vi "DecodificaDO.vi"(0 "Array":T7[](array[typedef]), 7 "DO PLCs in":T5, 9 "statoDO Cdaq in":T9, 11 "DO interfaccia in":T6) -> (6 "Exit?":bool, 8 "DO PLCs out":T4, 10 "statoDO Cdaq out":T9, 15 "DO interfaccia out":T6)   [LabVIEW 2019]
uses:
  controls/statoDO_Cdaq.ctl
  SET SINGLE DO.ctl
  DO List.ctl
  TypeDef/DOinterfaccia.ctl
  ST1200_LIST_IO/StatoDO_PLC_1.ctl
  ST1200_LIST_IO/StatoDO_PLC_2.ctl
  ST1200_LIST_IO/StatoDO_PLC_3.ctl
  GlobalForzaUscite.vi
  Global_DO_Interfaccia.vi
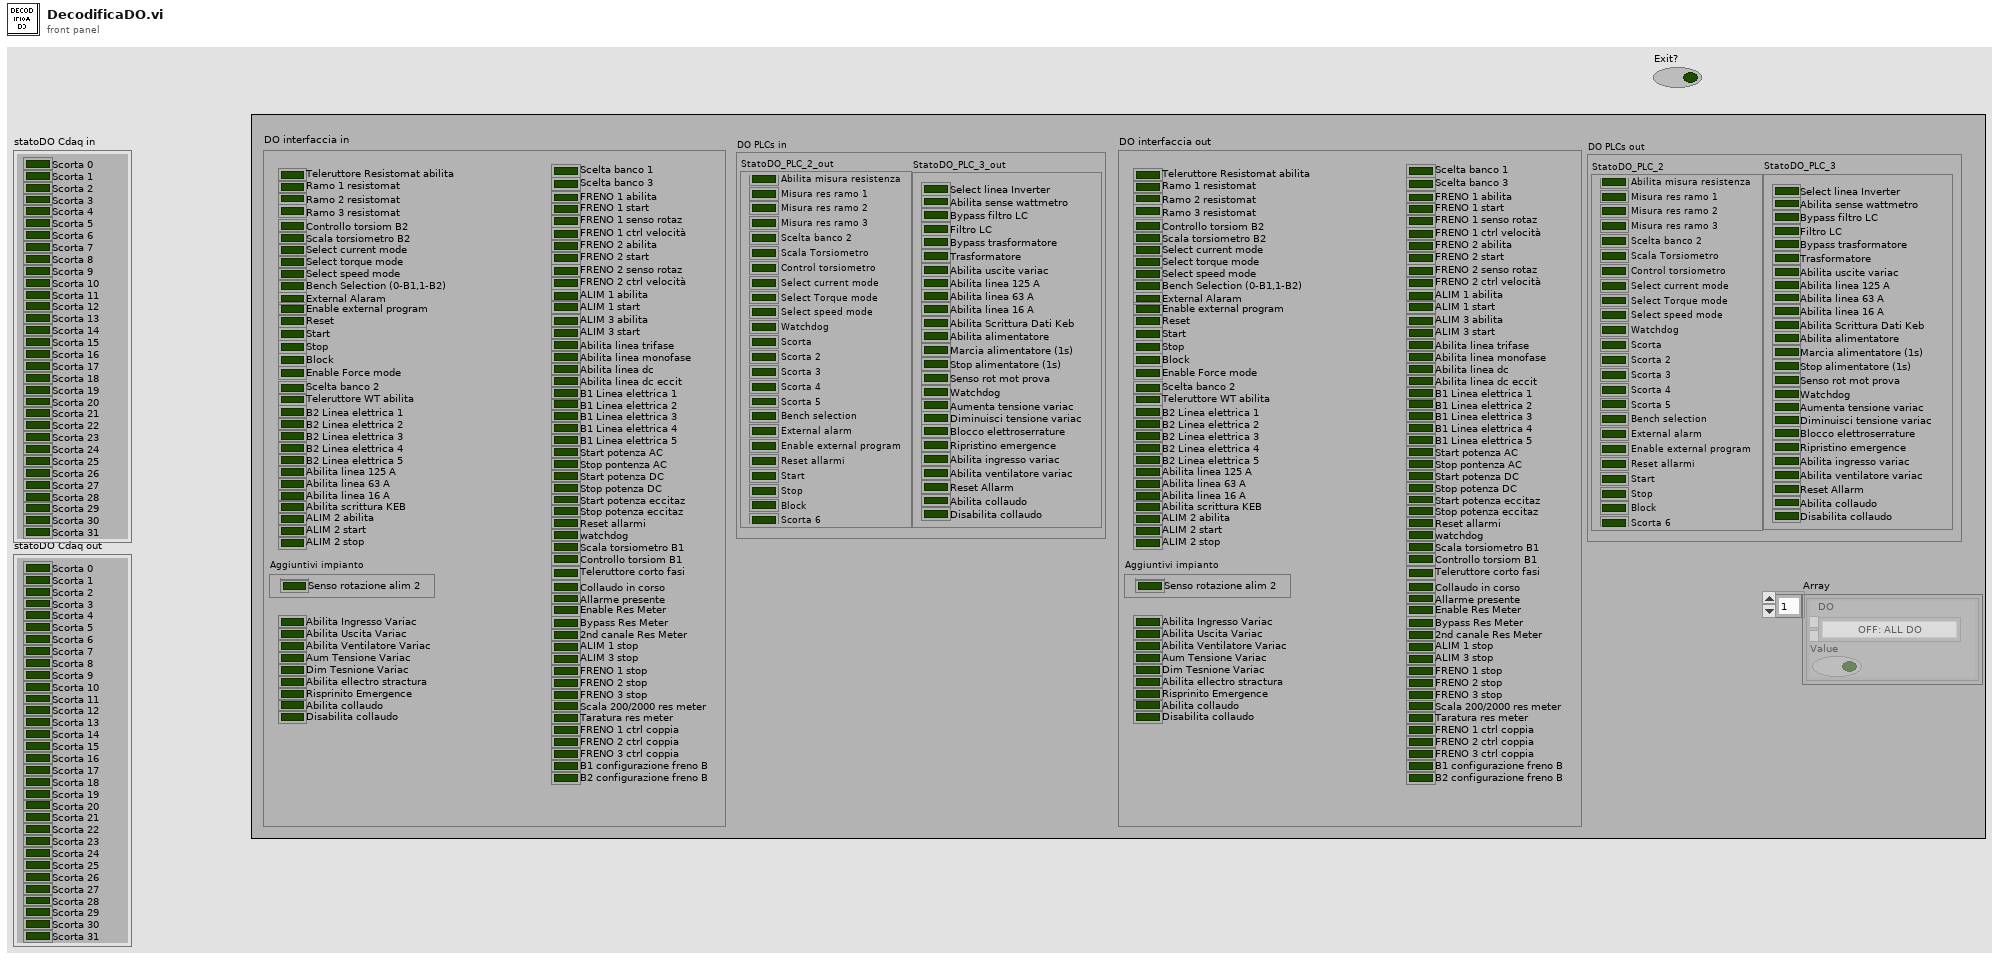
[diagram p1: front panel]
types:
  T1 = typedef "StatoDO_PLC_1.ctl" = cluster{"Scelta banco 1":bool, "Set dati motore freno 2":bool, "Diretto inverter":bool, "Filtro LC":bool, "Marcia ALIM (1s)":bool, "Marcia FRENO (1s)":bool, "Stop AFE (1s)":bool, "Stop freno (1s)":bool, "Reset allarmi":bool, "Watchdog":bool, "Senso rotazione":bool, "Abilita collaudo (1s)":bool, "Disabilita collaudo (1s)":bool, "Abilitazione ALIM":bool, "Abilitazione FRENO":bool, "Teleruttore WT":bool, "Senso rot motore prova":bool, "Scorta 7":bool, "Scorta 8":bool, "Scorta 9":bool, "Scorta 10":bool, "Scorta 11":bool, "Scorta 12":bool, "Scorta 13":bool}
  T2 = typedef "StatoDO_PLC_2.ctl" = cluster{"Relè misura resistomat":bool, "Misura res ramo 1":bool, "Misura res ramo 2":bool, "Misura res ramo 3":bool, "Scelta banco 2":bool, "Scala Torsiometro":bool, "Ctrl torsiometro":bool, "Select current mode":bool, "Select Torque mode":bool, "Select speed mode":bool, "Watchdog":bool, "Scorta":bool, "Scorta 2":bool, "Scorta 3":bool, "Scorta 4":bool, "Scorta 5":bool, "Bench selection":bool, "External alarm":bool, "Enable external program":bool, "Reset allarmi":bool, "Start":bool, "Stop":bool, "Block":bool, "Scorta 6":bool}
  T3 = typedef "StatoDO_PLC_3.ctl" = cluster{"Select linea Inverter":bool, "Abilita sense wattmetro":bool, "Bypass filtro LC":bool, "Filtro LC":bool, "Bypass trasformatore":bool, "Trasformatore":bool, "Abilita uscite variac":bool, "Abilita linea 125 A":bool, "Abilita linea 63 A":bool, "Abilita linea 16 A":bool, "Abilita Scrittura Dati Keb":bool, "Abilita alimentatore":bool, "Marcia alimentatore (1s)":bool, "Stop alimentatore (1s)":bool, "Senso rot mot prova":bool, "Watchdog":bool, "Aumenta tensione variac":bool, "Diminuisci tensione variac ":bool, "Blocco elettroserrature":bool, "Ripristino emergence":bool, "Abilita ingresso variac":bool, "Abilita ventilatore variac":bool, "Reset Allarm":bool, "Scorta 1":bool, "Scorta 2":bool, "Scorta 3":bool, "Scorta 4":bool, "Scorta 5":bool, "Scorta 6":bool, "Scorta 7":bool, "Scorta 8":bool, "Scorta 9":bool, "Abilita collaudo":bool, "Disabilita collaudo ":bool, "Scorta 10":bool, "Scorta 11":bool, "Scorta 12":bool, "Scorta 13":bool, "Scorta 14":bool, "Scorta 15":bool}
  T4 = cluster{"StatoDO_PLC 1":T1, "StatoDO_PLC_2":T2, "StatoDO_PLC_3":T3}
  T5 = cluster{"StatoDO_PLC 1 in":T1, "StatoDO_PLC_2_out":T2, "StatoDO_PLC_3_out":T3}
  T6 = typedef "DOinterfaccia.ctl" = cluster{"Scelta banco 1":bool, "Scelta banco 2":bool, "Scelta banco 3":bool, "FRENO 1 abilita":bool, "FRENO 1 start":bool, "FRENO 1 senso rotaz":bool, "FRENO 1 ctrl velocità":bool, "FRENO 2 abilita":bool, "FRENO 2 start":bool, "FRENO 2 senso rotaz":bool, "FRENO 2 ctrl velocità":bool, "ALIM 1 abilita":bool, "ALIM 1 start":bool, "ALIM 2 abilita":bool, "ALIM 2 start":bool, "ALIM 3 abilita":bool, "ALIM 3 start":bool, "Abilita linea trifase":bool, "Abilita linea monofase":bool, "Abilita linea dc":bool, "Abilita linea dc eccit":bool, "B1 Linea elettrica 1":bool, "B1 Linea elettrica 2":bool, "B1 Linea elettrica 3":bool, "B1 Linea elettrica 4":bool, "B1 Linea elettrica 5":bool, "B2 Linea elettrica 1":bool, "B2 Linea elettrica 2":bool, "B2 Linea elettrica 3":bool, "B2 Linea elettrica 4":bool, "B2 Linea elettrica 5":bool, "Start potenza AC":bool, "Stop pontenza AC":bool, "Start potenza DC":bool, "Stop potenza DC":bool, "Start potenza eccitaz":bool, "Stop potenza eccitaz":bool, "Reset allarmi":bool, "watchdog":bool, "Scala torsiometro B1":bool, "Controllo torsiom B1":bool, "Scala torsiometro B2":bool, "Controllo torsiom B2":bool, "Teleruttore WT abilita":bool, "Teleruttore Resistomat abilita":bool, "Teleruttore corto fasi":bool, "Ramo 1 resistomat":bool, "Ramo 2 resistomat":bool, "Ramo 3 resistomat":bool, "Collaudo in corso":bool, "Allarme presente":bool, "Enable Res Meter":bool, "Bypass Res Meter":bool, "2nd canale Res Meter":bool, "Scala 200/2000 res meter":bool, "Taratura res meter":bool, "FRENO 1 ctrl coppia":bool, "FRENO 2 ctrl coppia":bool, "FRENO 3 ctrl coppia":bool, "Aggiuntivi impianto":cluster{"Senso rotazione alim 1":bool, "Senso rotazione alim 2":bool}, "ALIM 1 stop":bool, "ALIM 2 stop":bool, "ALIM 3 stop":bool, "FRENO 1 stop":bool, "FRENO 2 stop":bool, "FRENO 3 stop":bool, "B1 configurazione freno B":bool, "B2 configurazione freno B":bool, "Abilita scrittura KEB":bool, "Bench Selection (0-B1,1-B2)":bool, "Select current mode":bool, "Select torque mode":bool, "Select speed mode":bool, "Start":bool, "Stop":bool, "Block":bool, "Enable Force mode":bool, "Abilita linea 125 A":bool, "Abilita linea 63 A":bool, "Abilita linea 16 A":bool, "Aum Tensione Variac":bool, "Dim Tesnione Variac":bool, "Abilita ellectro stractura":bool, "Risprinito Emergence":bool, "Abilita collaudo":bool, "Disabilita collaudo":bool, "External Alaram":bool, "Enable external program":bool, "Reset":bool, "Abilita Ingresso Variac":bool, "Abilita Ventilatore Variac":bool, "Abilita Uscita Variac ":bool}
  T7 = typedef "SET SINGLE DO.ctl" = cluster{"DO":T8, "Value":bool}
  T8 = typedef "DO List.ctl" = enum16{"OFF: ALL DO", "*ABILITA freno 1", "*ABILITA freno 2", "*ABILITA freno 3", "*START freno 1", "*START freno 2", "*START freno 3", "*STOP freno 1", "*STOP freno 3", "*STOP freno 2", "*Senso rot freno 1", "*Senso rot freno 2", "*Senso rot freno 3", "*Ctrl velocità freno 1", "*Ctrl velocità freno 2", "*Ctrl velocità freno 3", "*Ctrl coppia freno 1", "*Ctrl coppia freno 2", "*Ctrl coppia freno 3", "*ABILITA alimentatore 1", "*ABILITA alimentatore 2", "*ABILITA alimentatore 3", "*ABILITA alimentatore 4", "*START alimentatore 1", "*START alimentatore 2", "*START alimentatore 3", "*START alimentatore 4", "*STOP alimentatore 1", "*STOP alimentatore 2", "*STOP alimentatore 3", "*STOP alimentatore 4", "SENSO ROT alimentatore 1", "SENSO ROT alimentatore 2", "Abilita LEM 1000A", "Abilita LEM 300A", "Abilita sensori EXT WT", "B1 Seleziona linea 1", "B1 Seleziona linea 2", "B1 Seleziona linea 3", "B1 Seleziona linea 4", "B1 Seleziona linea 5", "B2 Seleziona linea 1", "B2 Seleziona linea 2", "B2 Seleziona linea 3", "B2 Seleziona linea 4", "B2 Seleziona linea 5", "*Reset allarmi", "*Start potenza AC", "*Stop potenza AC", "*Start potenza DC", "*Stop potenza DC", "*Start potenza DC eccit", "*Stop pontenza DC eccit", "Bypass res meter", "2nd canale res meter", "Enable res meter", "*Abilit teler ramo WT", "*Abil teler ramo princ Resit", "*Abil teler ramo 1 Resist", "*Abil teler ramo 2 Resist", "*Abil teler ramo 3 Resist", "*Abil cortocirc avvolgim", "*Controllo torsiometro B1", "*Controllo Torsiom B2", "*Scala torsiometro B1", "*Scala torsiometro B2", "*Collaudo in corso", "*Allarme presente", "Abilitazione elettroserratura", "Exit", "*Abilita collaudo", "*Abilita potenza trifase", "*Abilita potenza monofase", "*Abilita potenza DC", "*Abilita potenza DC eccit", "*Disabilita teleruttori potenza", "Set teleruttori prova a freddo", "Prova a freddo monofase", "Watchdog", "Forza DO PLC 3", "Forza DO PLC 2", "Forza DO PLC 1", "Forza DO cDAQ", "Scala 2000(T) 200(F) res meter", "Seleziona banco 1", "Seleziona banco 2", "Comando azionam in blocco", "Comando azionam reset", "Sensibilità freno 16 32 nm", "Reset Allarmi", "Carico res - Ramo 1", "Carico res - Ramo 2", "Carico res - Ramo 3", "Carico res - Ramo 4", "Carico res - Ramo 5", "Carico res - Ramo 6", "Carico res - Ramo 7", "Carico res - Ramo 8", "Carico res - Ramo 9", "Carico res - Ramo 10", "Carico res - Ramo 11", "Carico res - Start ventilatore", "Carico res - Stop ventilatore", "Abilita potenza solo freno", "Abilita AFE + freno trasc", "Abilita potenza carico resistivo", "Chiudi potenza AFE", "Apri potenza AFE", "Start AFE", "Config Banco2 TDE", "Misura diretto WT", "Ripristina centralina protezioni", "Abilita Scrittura Dati Keb", "Bench Selection(0-B1,1-B2)", "Select current mode", "Select torque mode", "Select speed mode", "Extenal alarm", "Enable Extenal program ", "Start ", "Stop", "Enable force mode", "Abilita linea 125 A", "Abilita linea 63 A", "Abilita linea 16 A", "Aum Tensione Variac", "Dim Tesnione Variac", "Abilita Ellecto Stractura", "Riprinto Emergenxe ", "Abilita Collaudo", "Disabilita Collaudo", "Abilita Ingresso Variac", "Abilita Uscita Variac", "Abilita ventilatore Variac"}
  T9 = typedef "statoDO_Cdaq.ctl" = cluster{"Scorta 0":bool, "Scorta 1":bool, "Scorta 2":bool, "Scorta 3":bool, "Scorta 4":bool, "Scorta 5":bool, "Scorta 6":bool, "Scorta 7":bool, "Scorta 8":bool, "Scorta 9":bool, "Scorta 10":bool, "Scorta 11":bool, "Scorta 12":bool, "Scorta 13":bool, "Scorta 14":bool, "Scorta 15":bool, "Scorta 16":bool, "Scorta 17":bool, "Scorta 18":bool, "Scorta 19":bool, "Scorta 20":bool, "Scorta 21":bool, "Scorta 22":bool, "Scorta 23":bool, "Scorta 24":bool, "Scorta 25":bool, "Scorta 26":bool, "Scorta 27":bool, "Scorta 28":bool, "Scorta 29":bool, "Scorta 30":bool, "Scorta 31":bool}
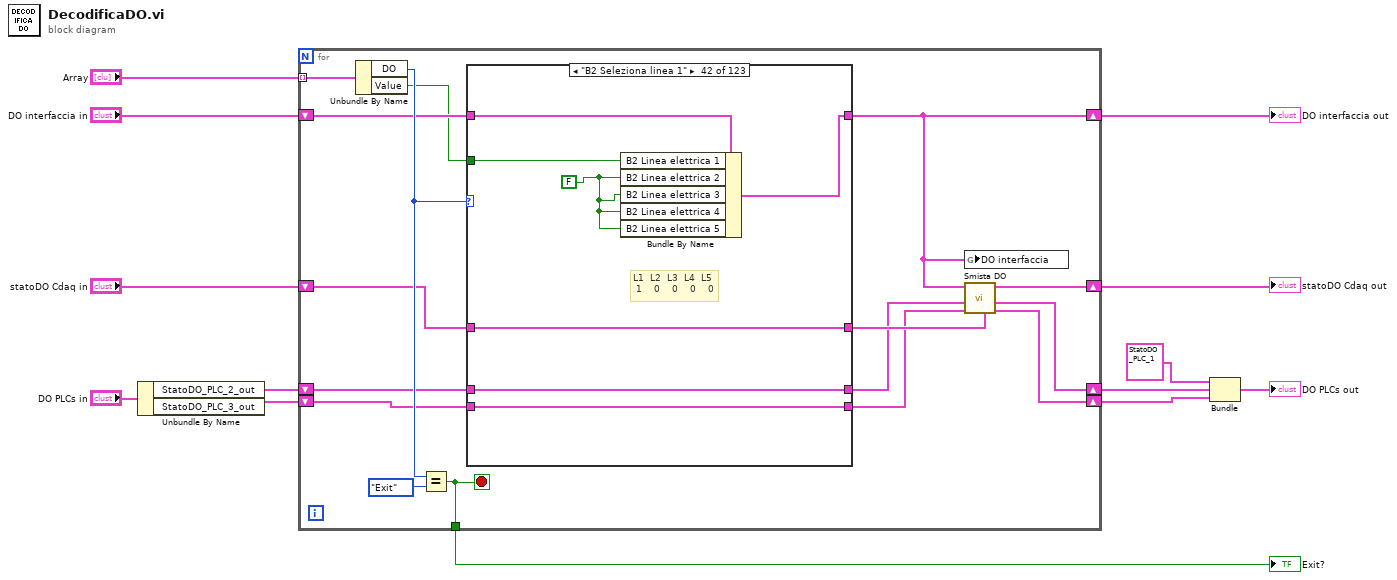
[diagram p0: block diagram]
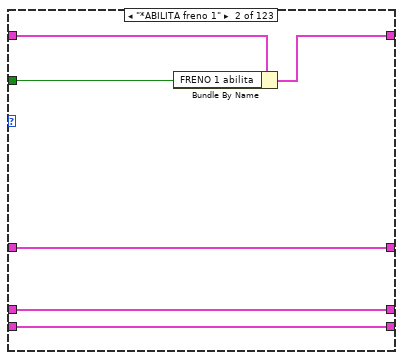
[diagram p3: hidden frame]
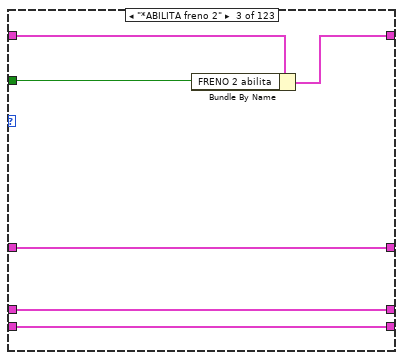
[diagram p4: hidden frame]
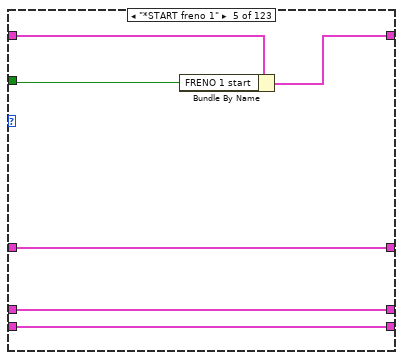
[diagram p6: hidden frame]
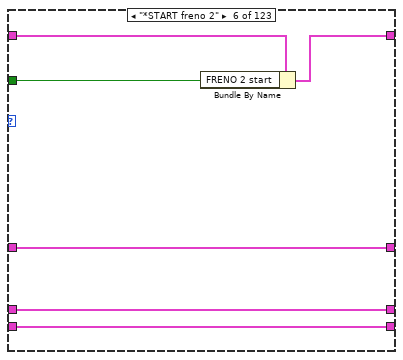
[diagram p7: hidden frame]
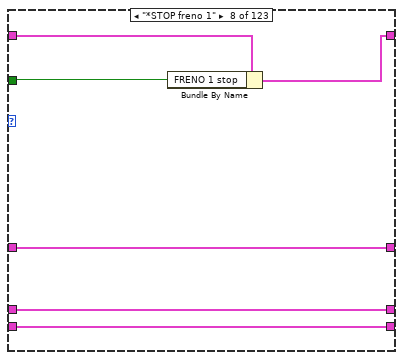
[diagram p9: hidden frame]
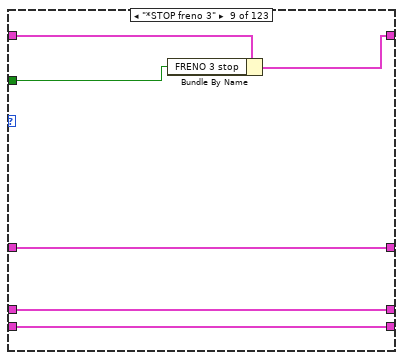
[diagram p10: hidden frame]
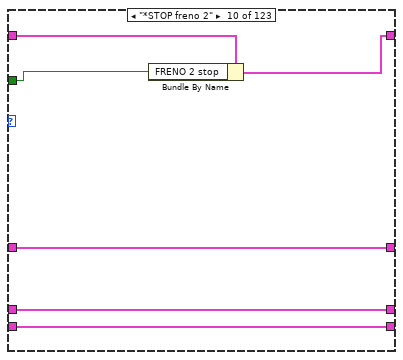
[diagram p11: hidden frame]
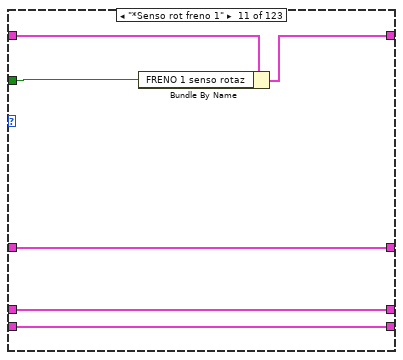
[diagram p12: hidden frame]
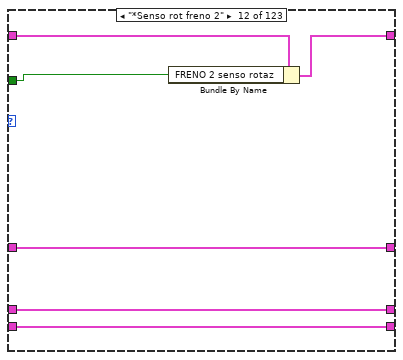
[diagram p13: hidden frame]
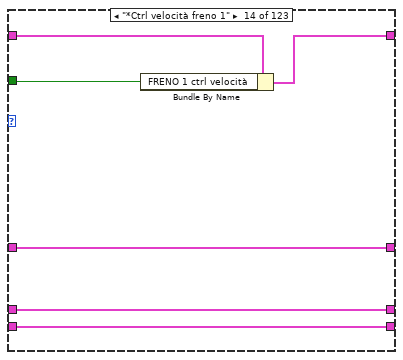
[diagram p15: hidden frame]
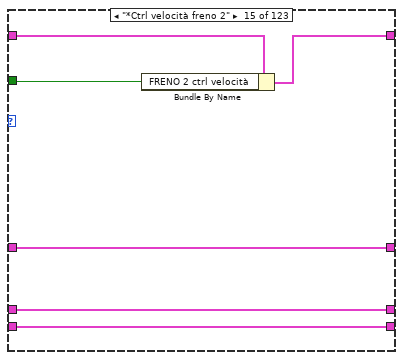
[diagram p16: hidden frame]
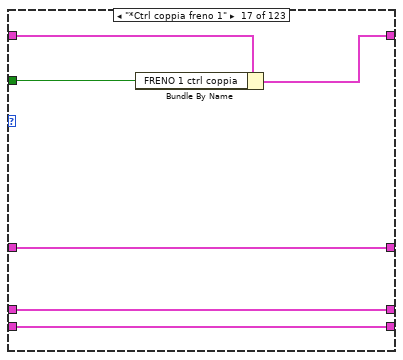
[diagram p18: hidden frame]
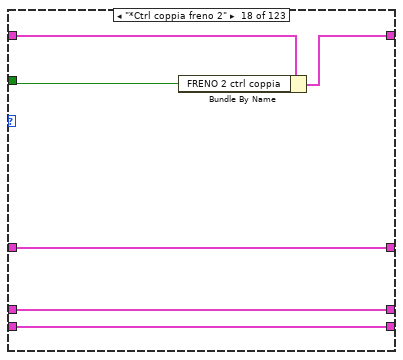
[diagram p19: hidden frame]
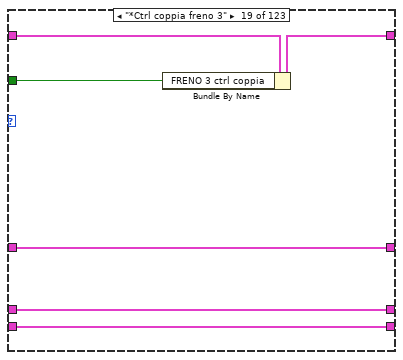
[diagram p20: hidden frame]
diagram:
  n1 = Unbundle By Name("DO PLCs in") -> ("StatoDO_PLC_2_out"=w6:T2, "StatoDO_PLC_3_out"=w5:T3)
  n2 = for {
    tunnel: "Array" -> [w29] mode=indexing
    shift-right: [w26] -> w10
    shift-left: "statoDO Cdaq in" -> [w21]
    tunnel: [w28] -> w13
    shift-right: [w20] -> w8
    shift-left: "DO interfaccia in" -> [w23]
    shift-right: [w19] -> w4
    shift-left: w6 -> [w16]
    shift-right: [w18] -> w3
    shift-left: w5 -> [w17]
    stop <- w28 stop-if-true
    n3 = Unbundle By Name(w29) -> ("DO"=w25:T8, "Value"=w22:bool)
    n4 = Equal?(x=w25, y=DO_List."Exit" ("DO")) -> (x = y?=w28:bool)
    n5 = case shown="\"B2 Seleziona linea 1\"" w25 {
      tunnel: [w32 w38 w44 w48 w54 w60 w64 w70 w76 w82 w88 w94 w98 w104 w110 w114 w120 w126 w132 w138 w144 w150 w154 w160 w166 w172 w176 w182 w188 w194 w198 w204 w210 w216 w220 w224 w231 w238 w245 w252 w259 w266 w273 w280 w287 w294 w300 w306 w312 w318 w324 w328 w332 w338 w344 w350 w356 w362 w368 w374 w380 w386 w392 w398 w404 w410 w416 w422 w426 w430 w434 w441 w448 w455 w462 w468 w475 w479 w485 w487 w493 w497 w498 w507 w513 w519 w523 w527 w531 w537 w541 w545 w549 w553 w557 w561 w565 w569 w573 w577 w581 w585 w589 w595 w599 w603 w607 w611 w615 w621 w627 w631 w637 w643 w649 w655 w661 w667 w673 w679 w685 w691 w697] -> w24
      tunnel: [_ w35 w42 w47 w51 w58 w63 w65 w72 w78 w86 w92 w97 w102 w108 w113 w117 w124 w130 w136 w142 w148 w153 w158 w164 w170 w175 w177 w183 w189 w197 w200 w206 w211 w217 w221 w229 w235 w243 w250 w257 w262 w269 w276 w283 w290 w298 w304 w308 w316 w320 w325 w329 w336 w342 w348 w354 w360 w366 w372 w378 w384 w389 w396 w402 w407 w414 w420 w423 w429 w433 w439 w444 w451 w458 w466 w473 w478 w483 w489 w492 w496 w501 w505 w511 w515 w520 w524 w528 w535 w538 w542 w546 w550 w554 w558 w562 w566 w570 w574 w578 w582 w586 w591 w596 w600 w604 w608 w612 w617 w623 w628 w632 w638 w645 w651 w657 w663 w669 w675 w681 w687 w693] -> w20
      tunnel: w23 -> [_ w37 w43 w47 w52 w59 w63 w67 w73 w79 w87 w93 w97 w103 w109 w113 w118 w125 w131 w137 w143 w149 w153 w159 w165 w171 w175 w179 w184 w190 w197 w201 w207 w212 w217 w221 w230 w236 w244 w251 w258 w263 w270 w277 w284 w291 w299 w305 w309 w317 w321 w325 w329 w337 w343 w349 w355 w361 w367 w373 w379 w385 w390 w397 w403 w408 w415 w421 w423 w429 w433 w440 w445 w452 w459 w467 w474 w478 w484 w489 w492 w496 w501 w506 w512 w516 w520 w524 w528 w536 w538 w542 w546 w550 w554 w558 w562 w566 w570 w574 w578 w582 w586 w592 w596 w600 w604 w608 w612 w618 w624 w628 w634 w640 w646 w652 w658 w664 w670 w676 w682 w688 w694]
      tunnel: w22 -> [_ w36 w41 _ w53 w57 _ w66 w71 w77 w85 w91 _ w101 w107 _ w119 w123 w129 w135 w141 w147 _ w157 w163 w169 _ w178 w185 w191 _ w199 w205 w213 _ _ w228 w237 w242 w249 w256 w261 w268 w275 w282 w288 w295 w303 w307 w315 w319 _ _ w335 w341 w347 w353 w359 w365 w371 w377 w383 w391 w395 w401 w409 w413 w419 _ _ _ w438 w443 w450 w457 _ _ _ w482 _ _ _ _ w504 w510 w514 _ _ _ w532 _ _ _ _ _ _ _ _ _ _ _ _ _ _ _ _ _ _ _ w616 w622 _ w633 w639 w644 w650 w656 w662 w668 w674 w680 w686 w692]
      tunnel: w21 -> [w32 w38 w44 w48 w54 w60 w64 w70 w76 w82 w88 w94 w98 w104 w110 w114 w120 w126 w132 w138 w144 w150 w154 w160 w166 w172 w176 w182 w188 w194 w198 w204 w210 w216 w220 w224 w231 w238 w245 w252 w259 w266 w273 w280 w287 w294 w300 w306 w312 w318 w324 w328 w332 w338 w344 w350 w356 w362 w368 w374 w380 w386 w392 w398 w404 w410 w416 w422 w426 w430 w434 w441 w448 w455 w462 w468 w475 w479 w485 w487 w493 w497 _ w507 w513 w519 w523 w527 w531 w537 w541 w545 w549 w553 w557 w561 w565 w569 w573 w577 w581 w585 w589 w595 w599 w603 w607 w611 w615 w621 w627 w631 w637 w643 w649 w655 w661 w667 w673 w679 w685 w691 w697]
      tunnel: w17 -> [w30 w33 w39 w45 w49 w55 w61 w68 w74 w80 w83 w89 w95 w99 w105 w111 w115 w121 w127 w133 w139 w145 w151 w155 w161 w167 w173 w180 w186 w192 w195 w202 w208 w214 w218 w222 w225 w232 w239 w246 w253 w264 w271 w278 w285 w292 w296 w301 w310 w313 w322 w326 w330 w333 w339 w345 w351 w357 w363 w369 w375 w381 w387 w393 w399 w405 w411 w417 w424 w427 w431 w436 w446 w453 w460 w464 w469 w476 w480 _ w491 w494 w499 w502 w508 w517 w521 w525 w529 w533 w539 w543 w547 w551 w555 w559 w563 w567 w571 w575 w579 w583 w587 w593 w597 w601 w605 w609 w613 w619 w625 w629 w635 w641 w647 w653 w659 w665 w671 w677 w683 w689 w695]
      tunnel: w16 -> [w31 w34 w40 w46 w50 w56 w62 w69 w75 w81 w84 w90 w96 w100 w106 w112 w116 w122 w128 w134 w140 w146 w152 w156 w162 w168 w174 w181 w187 w193 w196 w203 w209 w215 w219 w223 w226 w233 w240 w247 w254 w265 w272 w279 w286 w293 w297 w302 w311 w314 w323 w327 w331 w334 w340 w346 w352 w358 w364 w370 w376 w382 w388 w394 w400 w406 w412 w418 w425 w428 w432 w437 w447 w454 w461 w465 w470 w477 w481 w488 _ w495 w500 w503 w509 w518 w522 w526 w530 w534 w540 w544 w548 w552 w556 w560 w564 w568 w572 w576 w580 w584 w588 w594 w598 w602 w606 w610 w614 w620 w626 w630 w636 w642 w648 w654 w660 w666 w672 w678 w684 w690 w696]
      tunnel: [w31 w34 w40 w46 w50 w56 w62 w69 w75 w81 w84 w90 w96 w100 w106 w112 w116 w122 w128 w134 w140 w146 w152 w156 w162 w168 w174 w181 w187 w193 w196 w203 w209 w215 w219 w223 w226 w233 w240 w247 w254 w265 w272 w279 w286 w293 w297 w302 w311 w314 w323 w327 w331 w334 w340 w346 w352 w358 w364 w370 w376 w382 w388 w394 w400 w406 w412 w418 w425 w428 w432 w437 w447 w454 w461 w465 w470 w477 w481 w488 w490 w495 w500 w503 w509 w518 w522 w526 w530 w534 w540 w544 w548 w552 w556 w560 w564 w568 w572 w576 w580 w584 w588 w594 w598 w602 w606 w610 w614 w620 w626 w630 w636 w642 w648 w654 w660 w666 w672 w678 w684 w690 w696] -> w15
      tunnel: [w30 w33 w39 w45 w49 w55 w61 w68 w74 w80 w83 w89 w95 w99 w105 w111 w115 w121 w127 w133 w139 w145 w151 w155 w161 w167 w173 w180 w186 w192 w195 w202 w208 w214 w218 w222 w225 w232 w239 w246 w253 w264 w271 w278 w285 w292 w296 w301 w310 w313 w322 w326 w330 w333 w339 w345 w351 w357 w363 w369 w375 w381 w387 w393 w399 w405 w411 w417 w424 w427 w431 w436 w446 w453 w460 w464 w469 w476 w480 w486 w491 w494 w499 w502 w508 w517 w521 w525 w529 w533 w539 w543 w547 w551 w555 w559 w563 w567 w571 w575 w579 w583 w587 w593 w597 w601 w605 w609 w613 w619 w625 w629 w635 w641 w647 w653 w659 w665 w671 w677 w683 w689 w695] -> w14
      frame "OFF: ALL DO", Default {
      }
      frame "*ABILITA freno 1" {
        n6 = Bundle By Name(cluster=w37, "FRENO 1 abilita"=w36) -> (w35:T6)
      }
      frame "*ABILITA freno 2" {
        n7 = Bundle By Name(cluster=w43, "FRENO 2 abilita"=w41) -> (w42:T6)
      }
      frame "*ABILITA freno 3" {
      }
      frame "*START freno 1" {
        n8 = Bundle By Name(cluster=w52, "FRENO 1 start"=w53) -> (w51:T6)
      }
      frame "*START freno 2" {
        n9 = Bundle By Name(cluster=w59, "FRENO 2 start"=w57) -> (w58:T6)
      }
      frame "*START freno 3" {
      }
      frame "*STOP freno 1" {
        n10 = Bundle By Name(cluster=w67, "FRENO 1 stop"=w66) -> (w65:T6)
      }
      frame "*STOP freno 3" {
        n11 = Bundle By Name(cluster=w73, "FRENO 3 stop"=w71) -> (w72:T6)
      }
      frame "*STOP freno 2" {
        n12 = Bundle By Name(cluster=w79, "FRENO 2 stop"=w77) -> (w78:T6)
      }
      frame "*Senso rot freno 1" {
        n13 = Bundle By Name(cluster=w87, "FRENO 1 senso rotaz"=w85) -> (w86:T6)
      }
      frame "*Senso rot freno 2" {
        n14 = Bundle By Name(cluster=w93, "FRENO 2 senso rotaz"=w91) -> (w92:T6)
      }
      frame "*Senso rot freno 3" {
      }
      frame "*Ctrl velocità freno 1" {
        n15 = Bundle By Name(cluster=w103, "FRENO 1 ctrl velocità"=w101) -> (w102:T6)
      }
      frame "*Ctrl velocità freno 2" {
        n16 = Bundle By Name(cluster=w109, "FRENO 2 ctrl velocità"=w107) -> (w108:T6)
      }
      frame "*Ctrl velocità freno 3" {
      }
      frame "*Ctrl coppia freno 1" {
        n17 = Bundle By Name(cluster=w118, "FRENO 1 ctrl coppia"=w119) -> (w117:T6)
      }
      frame "*Ctrl coppia freno 2" {
        n18 = Bundle By Name(cluster=w125, "FRENO 2 ctrl coppia"=w123) -> (w124:T6)
      }
      frame "*Ctrl coppia freno 3" {
        n19 = Bundle By Name(cluster=w131, "FRENO 3 ctrl coppia"=w129) -> (w130:T6)
      }
      frame "*ABILITA alimentatore 1" {
        n20 = Bundle By Name(cluster=w137, "ALIM 1 abilita"=w135) -> (w136:T6)
      }
      frame "*ABILITA alimentatore 2" {
        n21 = Bundle By Name(cluster=w143, "ALIM 2 abilita"=w141) -> (w142:T6)
      }
      frame "*ABILITA alimentatore 3" {
        n22 = Bundle By Name(cluster=w149, "ALIM 3 abilita"=w147) -> (w148:T6)
      }
      frame "*ABILITA alimentatore 4" {
      }
      frame "*START alimentatore 1" {
        n23 = Bundle By Name(cluster=w159, "ALIM 1 start"=w157) -> (w158:T6)
      }
      frame "*START alimentatore 2" {
        n24 = Bundle By Name(cluster=w165, "ALIM 2 start"=w163) -> (w164:T6)
      }
      frame "*START alimentatore 3" {
        n25 = Bundle By Name(cluster=w171, "ALIM 3 start"=w169) -> (w170:T6)
      }
      frame "*START alimentatore 4" {
      }
      frame "*STOP alimentatore 1" {
        n26 = Bundle By Name(cluster=w179, "ALIM 1 stop"=w178) -> (w177:T6)
      }
      frame "*STOP alimentatore 2" {
        n27 = Bundle By Name(cluster=w184, "ALIM 2 stop"=w185) -> (w183:T6)
      }
      frame "*STOP alimentatore 3" {
        n28 = Bundle By Name(cluster=w190, "ALIM 3 stop"=w191) -> (w189:T6)
      }
      frame "*STOP alimentatore 4" {
      }
      frame "SENSO ROT alimentatore 1" {
        n29 = Bundle By Name(cluster=w201, "Aggiuntivi impianto.Senso rotazione alim 1"=w199) -> (w200:T6)
      }
      frame "SENSO ROT alimentatore 2" {
        n30 = Bundle By Name(cluster=w207, "Aggiuntivi impianto.Senso rotazione alim 2"=w205) -> (w206:T6)
      }
      frame "Abilita LEM 1000A" {
        n31 = Bundle By Name(cluster=w212, "Aggiuntivi impianto.Senso rotazione alim 2"=w213) -> (w211:T6)
      }
      frame "Abilita LEM 300A" {
      }
      frame "Abilita sensori EXT WT" {
      }
      frame "B1 Seleziona linea 1" {
        w227 = FALSE ("Linea elettrica 5")
        n32 = Bundle By Name(cluster=w230, "B1 Linea elettrica 1"=w228, "B1 Linea elettrica 2"=w227, "B1 Linea elettrica 3"=w227, "B1 Linea elettrica 4"=w227, "B1 Linea elettrica 5"=w227) -> (w229:T6)
      }
      frame "B1 Seleziona linea 2" {
        w234 = FALSE ("Linea elettrica 1")
        n33 = Bundle By Name(cluster=w236, "B1 Linea elettrica 1"=w234, "B1 Linea elettrica 2"=w237, "B1 Linea elettrica 3"=w234, "B1 Linea elettrica 4"=w234, "B1 Linea elettrica 5"=w234) -> (w235:T6)
      }
      frame "B1 Seleziona linea 3" {
        w241 = FALSE ("Linea elettrica 1")
        n34 = Bundle By Name(cluster=w244, "B1 Linea elettrica 1"=w241, "B1 Linea elettrica 2"=w241, "B1 Linea elettrica 3"=w242, "B1 Linea elettrica 4"=w241, "B1 Linea elettrica 5"=w241) -> (w243:T6)
      }
      frame "B1 Seleziona linea 4" {
        w248 = FALSE ("Linea elettrica 5")
        n35 = Bundle By Name(cluster=w251, "B1 Linea elettrica 1"=w248, "B1 Linea elettrica 2"=w248, "B1 Linea elettrica 3"=w248, "B1 Linea elettrica 4"=w249, "B1 Linea elettrica 5"=w248) -> (w250:T6)
      }
      frame "B1 Seleziona linea 5" {
        w255 = FALSE ("Linea elettrica 1")
        n36 = Bundle By Name(cluster=w258, "B1 Linea elettrica 1"=w255, "B1 Linea elettrica 2"=w255, "B1 Linea elettrica 3"=w255, "B1 Linea elettrica 4"=w255, "B1 Linea elettrica 5"=w256) -> (w257:T6)
      }
      frame "B2 Seleziona linea 1" {
        w260 = FALSE
        # "L1  L2  L3  L4  L5\n 1    0    0    0    0"
        n37 = Bundle By Name(cluster=w263, "B2 Linea elettrica 1"=w261, "B2 Linea elettrica 2"=w260, "B2 Linea elettrica 3"=w260, "B2 Linea elettrica 4"=w260, "B2 Linea elettrica 5"=w260) -> (w262:T6)
      }
      frame "B2 Seleziona linea 2" {
        w267 = FALSE ("B1 Linea elettrica 2")
        # "L1  L2  L3  L4  L5\n 0    1    0    0    0"
        n38 = Bundle By Name(cluster=w270, "B2 Linea elettrica 1"=w267, "B2 Linea elettrica 2"=w268, "B2 Linea elettrica 3"=w267, "B2 Linea elettrica 4"=w267, "B2 Linea elettrica 5"=w267) -> (w269:T6)
      }
      frame "B2 Seleziona linea 3" {
        w274 = FALSE ("B1 Linea elettrica 2")
        # "L1  L2  L3  L4  L5\n 0    0    1    0    0"
        n39 = Bundle By Name(cluster=w277, "B2 Linea elettrica 1"=w274, "B2 Linea elettrica 2"=w274, "B2 Linea elettrica 3"=w275, "B2 Linea elettrica 4"=w274, "B2 Linea elettrica 5"=w274) -> (w276:T6)
      }
      frame "B2 Seleziona linea 4" {
        w281 = FALSE ("B1 Linea elettrica 2")
        # "L1  L2  L3  L4  L5\n 0    0    0    1    0"
        n40 = Bundle By Name(cluster=w284, "B2 Linea elettrica 1"=w281, "B2 Linea elettrica 2"=w281, "B2 Linea elettrica 3"=w281, "B2 Linea elettrica 4"=w282, "B2 Linea elettrica 5"=w281) -> (w283:T6)
      }
      frame "B2 Seleziona linea 5" {
        w289 = FALSE ("B1 Linea elettrica 2")
        # "L1  L2  L3  L4  L5\n 0    0    0    0    1"
        n41 = Bundle By Name(cluster=w291, "B2 Linea elettrica 1"=w289, "B2 Linea elettrica 2"=w289, "B2 Linea elettrica 3"=w289, "B2 Linea elettrica 4"=w289, "B2 Linea elettrica 5"=w288) -> (w290:T6)
      }
      frame "*Reset allarmi" {
        n42 = Bundle By Name(cluster=w299, "Reset allarmi"=w295) -> (w298:T6)
      }
      frame "*Start potenza AC" {
        n43 = Bundle By Name(cluster=w305, "Start potenza AC"=w303) -> (w304:T6)
      }
      frame "*Stop potenza AC" {
        n44 = Bundle By Name(cluster=w309, "Stop pontenza AC"=w307) -> (w308:T6)
      }
      frame "*Start potenza DC" {
        n45 = Bundle By Name(cluster=w317, "Start potenza DC"=w315) -> (w316:T6)
      }
      frame "*Stop potenza DC" {
        n46 = Bundle By Name(cluster=w321, "Stop potenza DC"=w319) -> (w320:T6)
      }
      frame "*Start potenza DC eccit" {
      }
      frame "*Stop pontenza DC eccit" {
      }
      frame "Bypass res meter" {
        n47 = Bundle By Name(cluster=w337, "Bypass Res Meter"=w335) -> (w336:T6)
      }
      frame "2nd canale res meter" {
        n48 = Bundle By Name(cluster=w343, "2nd canale Res Meter"=w341) -> (w342:T6)
      }
      frame "Enable res meter" {
        n49 = Bundle By Name(cluster=w349, "Enable Res Meter"=w347) -> (w348:T6)
      }
      frame "*Abilit teler ramo WT" {
        n50 = Bundle By Name(cluster=w355, "Teleruttore WT abilita"=w353) -> (w354:T6)
      }
      frame "*Abil teler ramo princ Resit" {
        n51 = Bundle By Name(cluster=w361, "Teleruttore Resistomat abilita"=w359) -> (w360:T6)
      }
      frame "*Abil teler ramo 1 Resist" {
        n52 = Bundle By Name(cluster=w367, "Ramo 1 resistomat"=w365) -> (w366:T6)
      }
      frame "*Abil teler ramo 2 Resist" {
        n53 = Bundle By Name(cluster=w373, "Ramo 2 resistomat"=w371) -> (w372:T6)
      }
      frame "*Abil teler ramo 3 Resist" {
        n54 = Bundle By Name(cluster=w379, "Ramo 3 resistomat"=w377) -> (w378:T6)
      }
      frame "*Abil cortocirc avvolgim" {
        n55 = Bundle By Name(cluster=w385, "Teleruttore corto fasi"=w383) -> (w384:T6)
      }
      frame "*Controllo torsiometro B1" {
        n56 = Bundle By Name(cluster=w390, "Controllo torsiom B1"=w391) -> (w389:T6)
      }
      frame "*Controllo Torsiom B2" {
        n57 = Bundle By Name(cluster=w397, "Controllo torsiom B2"=w395) -> (w396:T6)
      }
      frame "*Scala torsiometro B1" {
        n58 = Bundle By Name(cluster=w403, "Scala torsiometro B1"=w401) -> (w402:T6)
      }
      frame "*Scala torsiometro B2" {
        n59 = Bundle By Name(cluster=w408, "Scala torsiometro B2"=w409) -> (w407:T6)
      }
      frame "*Collaudo in corso" {
        n60 = Bundle By Name(cluster=w415, "Collaudo in corso"=w413) -> (w414:T6)
      }
      frame "*Allarme presente" {
        n61 = Bundle By Name(cluster=w421, "Allarme presente"=w419) -> (w420:T6)
      }
      frame "Abilitazione elettroserratura" {
      }
      frame "Exit" {
      }
      frame "*Abilita collaudo" {
      }
      frame "*Abilita potenza trifase" {
        w435 = FALSE ("Abilita linea monofase")
        n62 = Bundle By Name(cluster=w440, "Abilita linea trifase"=w438, "Abilita linea monofase"=w435, "Abilita linea dc"=w435, "Abilita linea dc eccit"=w435) -> (w439:T6)
      }
      frame "*Abilita potenza monofase" {
        w442 = FALSE ("Abilita linea trifase")
        n63 = Bundle By Name(cluster=w445, "Abilita linea trifase"=w442, "Abilita linea monofase"=w443, "Abilita linea dc"=w442, "Abilita linea dc eccit"=w442) -> (w444:T6)
      }
      frame "*Abilita potenza DC" {
        w449 = FALSE ("Abilita linea trifase")
        n64 = Bundle By Name(cluster=w452, "Abilita linea trifase"=w449, "Abilita linea monofase"=w449, "Abilita linea dc"=w450, "Abilita linea dc eccit"=w449) -> (w451:T6)
      }
      frame "*Abilita potenza DC eccit" {
        w456 = FALSE ("Aggiuntivi impianto.Abilita carico resistivo")
        n65 = Bundle By Name(cluster=w459, "Abilita linea trifase"=w456, "Abilita linea monofase"=w456, "Abilita linea dc"=w456, "Abilita linea dc eccit"=w457) -> (w458:T6)
      }
      frame "*Disabilita teleruttori potenza" {
        w463 = FALSE ("Start potenza AC")
        n66 = Bundle By Name(cluster=w467, "Start potenza AC"=w463, "Stop pontenza AC"=w463, "Start potenza DC"=w463, "Stop potenza DC"=w463, "Start potenza eccitaz"=w463, "Stop potenza eccitaz"=w463, "Abilita linea trifase"=w463, "Abilita linea monofase"=w463, "Abilita linea dc"=w463, "Abilita linea dc eccit"=w463) -> (w466:T6)
      }
      frame "Set teleruttori prova a freddo" {
        n67 = Bundle By Name(cluster=w474, "Teleruttore Resistomat abilita"=TRUE, "Teleruttore WT abilita"=FALSE) -> (w473:T6)
      }
      frame "Prova a freddo monofase" {
      }
      frame "Watchdog" {
        n68 = Bundle By Name(cluster=w484, "watchdog"=w482) -> (w483:T6)
      }
      frame "Forza DO PLC 3" {
        n69 = global read "GlobalForzaUscite.vi" "Forza DO plc 3"() -> (w486:T3)
      }
      frame "Forza DO PLC 2" {
        n70 = global read "GlobalForzaUscite.vi" "Forza DO plc 2"() -> (w490:T2)
      }
      frame "Forza DO PLC 1" {
      }
      frame "Forza DO cDAQ" {
        n71 = global read "GlobalForzaUscite.vi" "ForzaDO_Cdaq"() -> (w498:T9)
      }
      frame "Scala 2000(T) 200(F) res meter" {
        n72 = Bundle By Name(cluster=w506, "Scala 200/2000 res meter"=w504) -> (w505:T6)
      }
      frame "Seleziona banco 1" {
        n73 = Bundle By Name(cluster=w512, "Scelta banco 1"=w510) -> (w511:T6)
      }
      frame "Seleziona banco 2" {
        n74 = Bundle By Name(cluster=w516, "Scelta banco 2"=w514) -> (w515:T6)
      }
      frame "Comando azionam in blocco" {
      }
      frame "Comando azionam reset" {
      }
      frame "Sensibilità freno 16 32 nm" {
      }
      frame "Reset Allarmi" {
        n75 = Bundle By Name(cluster=w536, "Reset allarmi"=w532) -> (w535:T6)
      }
      frame "Carico res - Ramo 1" {
      }
      frame "Carico res - Ramo 2" {
      }
      frame "Carico res - Ramo 3" {
      }
      frame "Carico res - Ramo 4" {
      }
      frame "Carico res - Ramo 5" {
      }
      frame "Carico res - Ramo 6" {
      }
      frame "Carico res - Ramo 7" {
      }
      frame "Carico res - Ramo 8" {
      }
      frame "Carico res - Ramo 9" {
      }
      frame "Carico res - Ramo 10" {
      }
      frame "Carico res - Ramo 11" {
      }
      frame "Carico res - Start ventilatore" {
      }
      frame "Carico res - Stop ventilatore" {
      }
      frame "Abilita potenza solo freno" {
        w590 = FALSE ("Abilita carico resistivo")
        n76 = Bundle By Name(cluster=w592, "Abilita linea trifase"=w590, "Abilita linea monofase"=w590, "Abilita linea dc"=w590, "Abilita linea dc eccit"=w590) -> (w591:T6)
      }
      frame "Abilita AFE + freno trasc" {
      }
      frame "Abilita potenza carico resistivo" {
      }
      frame "Chiudi potenza AFE" {
      }
      frame "Apri potenza AFE" {
      }
      frame "Start AFE" {
      }
      frame "Config Banco2 TDE" {
        n77 = Bundle By Name(cluster=w618, "B1 configurazione freno B"=w616, "B2 configurazione freno B"=w616) -> (w617:T6)
      }
      frame "Misura diretto WT" {
        n78 = Bundle By Name(cluster=w624, "Aggiuntivi impianto.Senso rotazione alim 1"=w622) -> (w623:T6)
      }
      frame "Ripristina centralina protezioni" {
      }
      frame "Abilita Scrittura Dati Keb" {
        n79 = Bundle By Name(cluster=w634, "Abilita scrittura KEB"=w633) -> (w632:T6)
      }
      frame "Bench Selection(0-B1,1-B2)" {
        n80 = Bundle By Name(cluster=w640, "Bench Selection (0-B1,1-B2)"=w639) -> (w638:T6)
      }
      frame "Select current mode" {
        n81 = Bundle By Name(cluster=w646, "Select current mode"=w644) -> (w645:T6)
      }
      frame "Select torque mode" {
        n82 = Bundle By Name(cluster=w652, "Select torque mode"=w650) -> (w651:T6)
      }
      frame "Select speed mode" {
        n83 = Bundle By Name(cluster=w658, "Select speed mode"=w656) -> (w657:T6)
      }
      frame "Abilita linea 125 A" {
        n84 = Bundle By Name(cluster=w664, "Abilita linea 125 A"=w662) -> (w663:T6)
      }
      frame "Abilita linea 63 A" {
        n85 = Bundle By Name(cluster=w670, "Abilita linea 63 A"=w668) -> (w669:T6)
      }
      frame "Abilita linea 16 A" {
        n86 = Bundle By Name(cluster=w676, "Abilita linea 16 A"=w674) -> (w675:T6)
      }
      frame "Aum Tensione Variac" {
        n87 = Bundle By Name(cluster=w682, "Aum Tensione Variac"=w680) -> (w681:T6)
      }
      frame "Dim Tesnione Variac" {
        n88 = Bundle By Name(cluster=w688, "Dim Tesnione Variac"=w686) -> (w687:T6)
      }
      frame "Abilita ventilatore Variac" {
        n89 = Bundle By Name(cluster=w694, "Abilita Ventilatore Variac"=w692) -> (w693:T6)
      }
    }
    n90 = global write "Global_DO_Interfaccia.vi" "DO interfaccia"(w20) -> ()
    n91 = call "Smista DO.vi"("Forza DO Cdaq"=w24, "Forza DO plc 3"=w14, "Forza DO plc 2"=w15, "DO interfaccia in"=w20) -> ("StatoDO_PLC_3_out"=w18:T3, "StatoDO_PLC_2_out"=w19:T2, "statoDO Cdaq out"=w26:T9)  [unwired: 5 in]
  }
  "statoDO Cdaq out" <- w10
  "Exit?" <- w13
  "DO interfaccia out" <- w8
  n92 = Bundle("StatoDO_PLC 1 in"=T1 {"Scelta banco 1"=FALSE, "Set dati motore freno 2"=FALSE, "Diretto inverter"=FALSE, "Filtro LC"=FALSE, "Marcia ALIM (1s)"=FALSE, "Marcia FRENO (1s)"=FALSE, "Stop AFE (1s)"=FALSE, "Stop freno (1s)"=FALSE, "Reset allarmi"=FALSE, "Watchdog"=FALSE, "Senso rotazione"=FALSE, "Abilita collaudo (1s)"=FALSE, "Disabilita collaudo (1s)"=FALSE, "Abilitazione ALIM"=FALSE, "Abilitazione FRENO"=FALSE, "Teleruttore WT"=FALSE, "Senso rot motore prova"=FALSE, "Scorta 7"=FALSE, "Scorta 8"=FALSE, "Scorta 9"=FALSE, "Scorta 10"=FALSE, "Scorta 11"=FALSE, "Scorta 12"=FALSE, "Scorta 13"=FALSE}, "StatoDO_PLC_2_out"=w4, "StatoDO_PLC_3_out"=w3) -> (→"DO PLCs out":T5)  [unwired: 1 in]
